vi "Get Setpoint.vi"(7 "Setpointindex":enum16{"Setpoint 1", "Setpoint 2", "Setpoint 3"}(ring), 8 "error in (no error)":errorcluster, 11 "VISA resource name":refnum<visa-resource-name>) -> (0 "error out":errorcluster, 1 "Setpoint (out)":dbl, 3 "VISA resource name out":refnum<visa-resource-name>)   [LabVIEW 2018, in "JULABO DeviceDriver.lvlib"]
doc: "This VI returns the actual value of the selected setpoint."
uses:
  JULABO DeviceDriver.lvlib
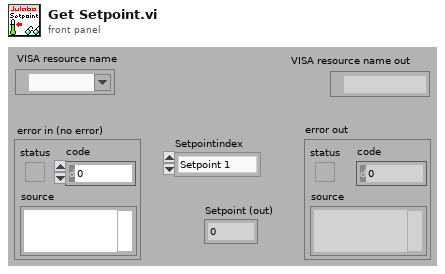
[diagram p1: front panel]
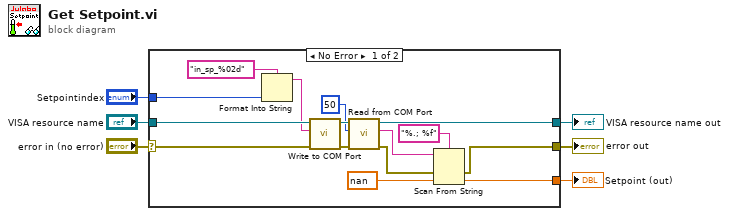
[diagram p0: block diagram]
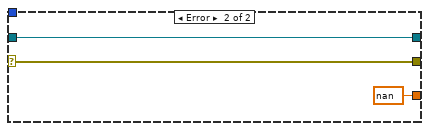
[diagram p2: hidden frame]
diagram:
  n1 = case shown="No Error" "error in (no error)" {
    selector: "error in (no error)" -> [w18 w23]
    tunnel: "VISA resource name" -> [w21 w24]
    tunnel: [w12 w23] -> w6
    tunnel: [w11 w24] -> w5
    tunnel: "Setpointindex" -> [w9 _]
    tunnel: [w8 nan ("Standardwert1")] -> w1
    frame No Error {
      n2 = Format Into String(format string="in_sp_%02d", w9) -> (resulting string=w19:string)  [unwired: 2 in, 1 out]
      n3 = call "Write to COM Port.vi"("error in"=w18, "Command (input)"=w19, "VISA resource name in"=w21) -> ("error out"=w17:errorcluster, "VISA resource name out"=w16:refnum<visa-resource-name>)  [unwired: 7 in]
      n4 = call "Read from COM Port.vi"("error in"=w17, "Byte to Read (-1:All)"=u32 50 ("Anzahl der Byte"), "VISA resource name in"=w16) -> ("error out"=w14:errorcluster, "String (output)"=w13:string, "VISA resource name out"=w11:refnum<visa-resource-name>)  [unwired: 5 in, 1 out]
      n5 = Scan From String(format string="%.; %f" ("Format-String"), input string=w13, error in=w14, default 1=nan ("Standardwert1")) -> (error out=w12:errorcluster, output 1=w8:dbl)  [unwired: 1 in, 2 out]
    }
    frame Error {
    }
  }
  "error out" <- w6
  "VISA resource name out" <- w5
  "Setpoint (out)" <- w1
